vi "Write tdms.vi"(0 "reference in":refnum<class "TDMS_DataHandler.lvclass">, 2 "Channel index to save":T1(array[ring]), 3 "Data in":waveform(dbl)[](array[waveform]), 5 "error in (no error)":errorcluster) -> (14 "reference out":refnum<class "TDMS_DataHandler.lvclass">, 15 "Channels to save out":string[](array[string]), 19 "error out":errorcluster)   [LabVIEW 2019, in "TDMS_DataHandler.lvclass"]
doc: "Writes raw data into tdms channels"
uses:
  TDMS_DataHandler.lvclass
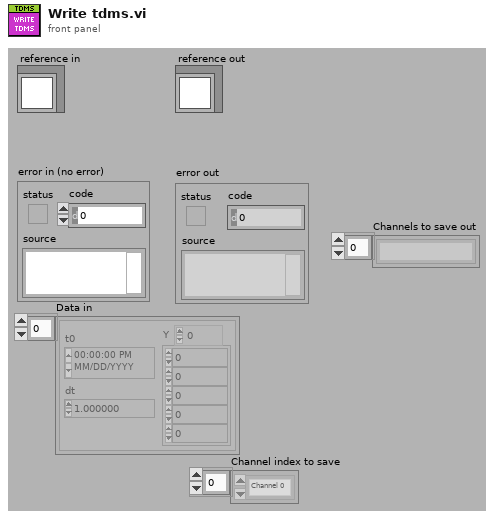
[diagram p1: front panel]
types:
  T1 = enum16{"Channel 0", "Channel 1", "Channel 2", "Channel 3"}[]
  T2 = typedef "TDMS_DataHandler.lvclass/ObjectAttributes.ctl" = cluster{"Directory":path, "FilePath":path, "FileRef":refnum<k34>, "ExperimentName":string, "GroupName":string, "ChannelNames":string[], "Datum":waveform(dbl)[], "Group_Metadata":cluster{"property names":string[], "property values":variant[]}, "Channel_Metadata":cluster{"property names":string[], "property values":variant[]}}
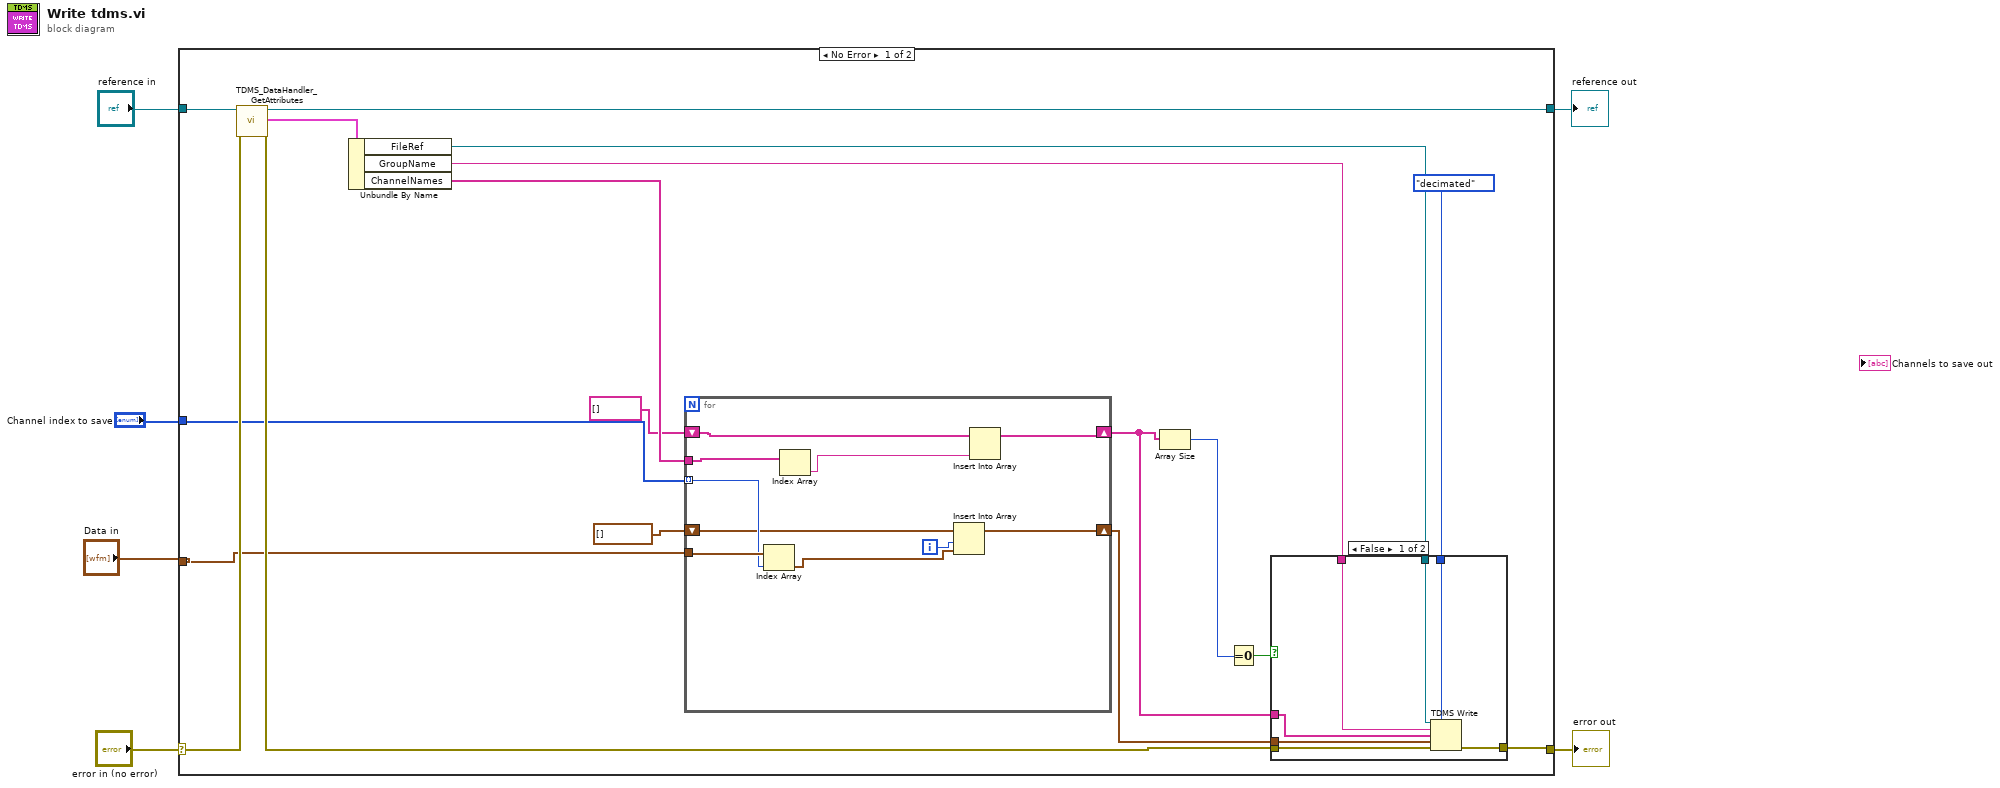
[diagram p0: block diagram]
diagram:
  n1 = case shown="No Error" "error in (no error)" {
    selector: "error in (no error)" -> [w24 w44]
    tunnel: [w19 w44] -> w5
    tunnel: [w23 w43] -> w3
    tunnel: "reference in" -> [w21 w43]
    tunnel: "Data in" -> [w15 _]
    tunnel: "Channel index to save" -> [w12 _]
    frame No Error {
      n2 = call "TDMS_DataHandler_GetAttributes.vi"("reference in"=w21, "error in (no error)"=w24) -> ("reference out"=w23:refnum<class "TDMS_DataHandler.lvclass">, "attributes"=w22:T2, "error out"=w20:errorcluster)  [unwired: 14 in, 1 out]
      n3 = Unbundle By Name(w22) -> ("FileRef"=w18:refnum<k34>, "GroupName"=w16:string, "ChannelNames"=w11:string[])
      n4 = for {
        tunnel: w12 -> [w41] mode=indexing
        tunnel: w15 -> [w42]
        shift-right: [w39] -> w13
        shift-left: waveform(dbl)[] [] ("element") -> [w40]
        tunnel: w11 -> [w37]
        shift-right: [w34] -> w7
        shift-left: string[] [] ("ChannelNames") -> [w36]
        i -> [w33]
        n5 = Index Array(array=w42, index=w41) -> (element=w38:waveform(dbl))
        n6 = Index Array(array=w37) -> (element=w35:string)  [unwired: 1 in]
        n7 = Insert Into Array(array=w40, index=w33, new element=w38) -> (w39:waveform(dbl)[])
        n8 = Insert Into Array(array=w36, new element=w35) -> (w34:string[])  [unwired: 1 in]
      }
      n9 = Array Size(array=w7) -> (size(s)=w9:i32)
      n10 = Equal To 0?(x=w9) -> (x = 0?=w8:bool)
      n11 = case shown="False" w8 {
        tunnel: w20 -> [w31 w32]
        tunnel: [w30 w32] -> w19
        tunnel: w18 -> [w29 _]
        tunnel: enum16{"decimated", "interleaved"}."decimated" ("data layout (0:decimated)") -> [w28 _]
        tunnel: w16 -> [w27 _]
        tunnel: w13 -> [w26 _]
        tunnel: w7 -> [w25 _]
        frame False {
          n12 = TDMS Write(0:w29, 1:w28, 5:w27, 7:w25, 9:w26, 11:w31) -> (15:w30:errorcluster)  [unwired: 3 out]
        }
        frame True {
          # "Dont save anything,\nno channels selected"
        }
      }
    }
    frame Error {
    }
  }
  "error out" <- w5
  "reference out" <- w3
